vi "RemoveUnexpectedMetrics.vi"(8 "error in (no error)":errorcluster, 9 "Startup Analysis Configuration":T4, 11 "data in":T1) -> (0 "error out":errorcluster)   [LabVIEW 2017, in "McsaStartupAnalysis.lvlib"]
uses:
  <vilib>/addons/InsightCM/Devices/Shared/Mcsa/McsaStartupAnalysis/McsaStartupAnalysis.lvlib
  <vilib>/addons/InsightCM/Devices/Shared/Mcsa/McsaStartupAnalysis/controls/Config.ctl
  <vilib>/addons/InsightCM/Devices/Shared/Mcsa/McsaStartupAnalysis/controls/Group.ctl
  <vilib>/addons/InsightCM/Devices/Shared/Mcsa/McsaStartupAnalysis/controls/ChannelForStartup.ctl
  <vilib>/addons/InsightCM/Devices/Shared/Mcsa/McsaStartupAnalysis/controls/StartupFeature.ctl
  <vilib>/addons/InsightCM/Devices/Shared/Mcsa/McsaStartupAnalysis/controls/MotorInfo.ctl
  <vilib>/addons/InsightCM/Devices/Shared/Common/FileFlow/controls/data_eventRef.ctl
  <vilib>/addons/InsightCM/Devices/Shared/Common/DataEvent/controls/EventReference.ctl
  <vilib>/addons/InsightCM/Devices/Shared/Common/DataEvent/controls/Event.ctl
  <vilib>/addons/InsightCM/MessageBus/Base/controls/DataEvent.ctl
  <vilib>/addons/InsightCM/MessageBus/Base/controls/KeyValuePair.ctl
  <vilib>/addons/InsightCM/Devices/Shared/Common/DataEvent/controls/DataSet.ctl
  <vilib>/addons/InsightCM/MessageBus/Base/controls/DataSetMetadata.ctl
  <vilib>/addons/InsightCM/MessageBus/Base/controls/TrendPoint.ctl
  <vilib>/addons/InsightCM/MessageBus/Base/controls/TrendAlarmUpdate.ctl
  <vilib>/addons/InsightCM/MessageBus/Base/controls/TrendAlarmTransition.ctl
  <vilib>/addons/PointValueMap/controls/PointMap.ctl
  <vilib>/addons/InsightCM/Utilities/PropertyHelpers/PropertyHelpers.lvlib
  <vilib>/addons/InsightCM/Devices/Shared/Common/DataEvent/DataEvent.lvlib
  <vilib>/addons/PointValueMap/PointValueMap.lvlib
  <vilib>/addons/InsightCM/Devices/Shared/Common/FileFlow/FileFlow.lvlib
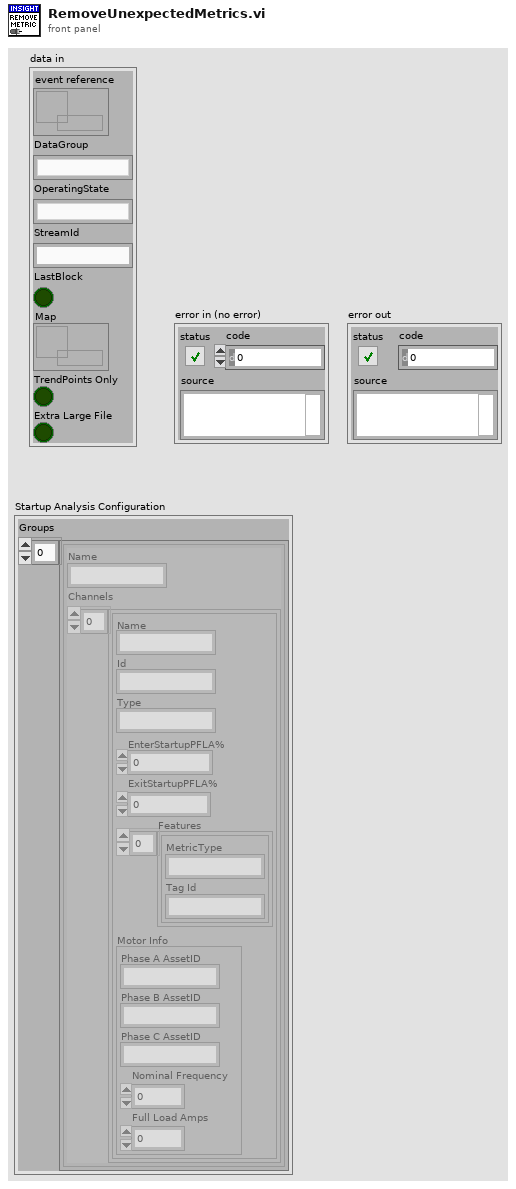
[diagram p1: front panel]
types:
  T1 = typedef "FileFlow.lvlib/data_eventRef.ctl" = cluster{"event reference":T2, "DataGroup":string, "OperatingState":string, "StreamId":string, "LastBlock":bool, "Map":T3, "TrendPoints Only":bool, "Extra Large File":bool}
  T2 = typedef "DataEvent.lvlib/EventReference.ctl" = refnum<data-value>
  T3 = typedef "PointValueMap.lvlib/PointMap.ctl" = refnum<data-value>
  T4 = typedef "McsaStartupAnalysis.lvlib/Config.ctl" = cluster{"Groups":T5[]}
  T5 = typedef "McsaStartupAnalysis.lvlib/Group.ctl" = cluster{"Name":string, "Channels":T6[]}
  T6 = typedef "McsaStartupAnalysis.lvlib/ChannelForStartup.ctl" = cluster{"Name":string, "Id":string, "Type":string, "EnterStartupPFLA%":dbl, "ExitStartupPFLA%":dbl, "Features":T7[], "Motor Info":T8}
  T7 = typedef "McsaStartupAnalysis.lvlib/StartupFeature.ctl" = cluster{"MetricType":string, "Tag Id":string}
  T8 = typedef "McsaStartupAnalysis.lvlib/MotorInfo.ctl" = cluster{"Phase A AssetID":string, "Phase B AssetID":string, "Phase C AssetID":string, "Nominal Frequency":dbl, "Full Load Amps":dbl}
  T9 = typedef "DataEvent.lvlib/Event.ctl" = cluster{"DataEvent":T10, "DataSets":T12[], "TrendPoints":T14[], "Alarms":T15[]}
  T10 = typedef "DataEvent.ctl" = cluster{"Id":string, "AssetNodeId":string, "Timestamp":i64, "Props":T11[]}
  T11 = typedef "KeyValuePair.ctl" = cluster{"Key":string, "Value":string}
  T12 = typedef "DataEvent.lvlib/DataSet.ctl" = cluster{"DataSetMetadata":T13, "Values":sgl[], "Values DVR":refnum<data-value>}
  T13 = typedef "DataSetMetadata.ctl" = cluster{"Id":string, "DataEventId":string, "AssetNodeId":string, "Type":string, "T0":i64, "Props":T11[]}
  T14 = typedef "TrendPoint.ctl" = cluster{"TrendPointId":string, "DataEventId":string, "Timestamp":i64, "Value":dbl, "Props":T11[]}
  T15 = typedef "TrendAlarmUpdate.ctl" = cluster{"RuleId":string, "Transition":T16}
  T16 = typedef "TrendAlarmTransition.ctl" = cluster{"At":i64, "Severity":i32, "Value":dbl}
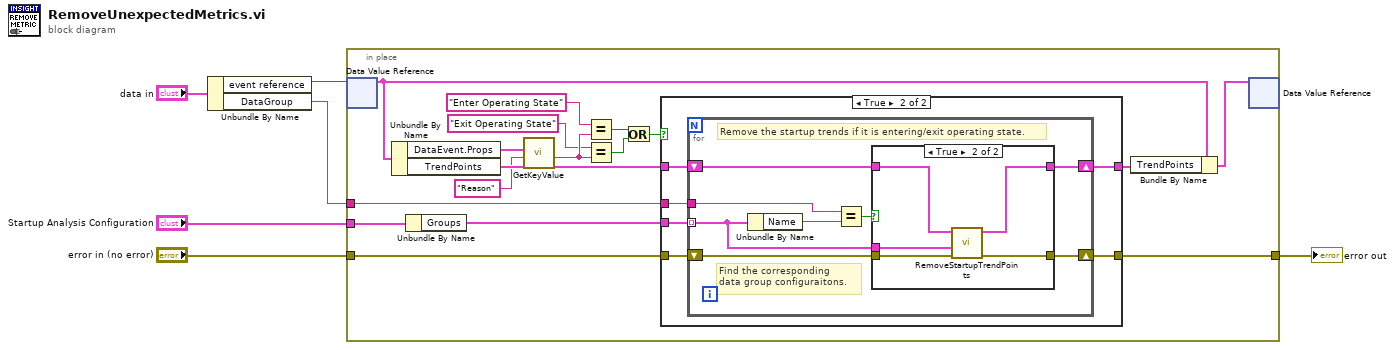
[diagram p0: block diagram]
diagram:
  n1 = Unbundle By Name("data in") -> ("event reference"=w4:T2, "DataGroup"=w3:string)
  n2 = in-place {
    in-place-border: "Startup Analysis Configuration" -> [w22]
    in-place-border: w3 -> [w17]
    in-place-border: "error in (no error)" -> [w16]
    in-place-border: [w15] -> w1
    n3 = in-place-dvr #1(w4) -> (w20:T9)  [unwired: 1 out]
    n4 = Unbundle By Name(w20) -> ("DataEvent.Props"=w14:T11[], "TrendPoints"=w19:T14[])
    n5 = Unbundle By Name(w22) -> ("Groups"=w23:T5[])
    n6 = call <vilib>:"GetKeyValue.vi"("key"="Reason" ("x"), "key value pairs"=w14) -> ("value"=w12:string)  [unwired: 7 in, 2 out]
    n7 = Equal?(x="Enter Operating State", y=w12) -> (x = y?=w9:bool)
    n8 = Equal?(x="Exit Operating State", y=w12) -> (x = y?=w8:bool)
    n9 = Or(x=w9, y=w8) -> (x .or. y?=w7:bool)
    n10 = case shown="True" w7 {
      tunnel: w23 -> [_ w31]
      tunnel: w19 -> [w25 w30]
      tunnel: [w25 w29] -> w18
      tunnel: w17 -> [_ w28]
      tunnel: w16 -> [w24 w27]
      tunnel: [w24 w26] -> w15
      frame False {
        # "Do nothing if it is not entering or exiting the operating state."
      }
      frame True {
        n11 = for {
          tunnel: w31 -> [w37] mode=indexing
          shift-right: [w35] -> w29
          shift-left: w30 -> [w36]
          tunnel: w28 -> [w34]
          shift-right: [w32] -> w26
          shift-left: w27 -> [w33]
          # "Remove the startup trends if it is entering/exit operating state."
          # "Find the corresponding\ndata group configuraitons."
          n12 = Unbundle By Name(w37) -> ("Name"=w39:string)
          n13 = Equal?(x=w34, y=w39) -> (x = y?=w38:bool)
          n14 = case shown="True" w38 {
            tunnel: w37 -> [_ w42]
            tunnel: w36 -> [w41 w46]
            tunnel: [w41 w45] -> w35
            tunnel: w33 -> [w40 w44]
            tunnel: [w40 w43] -> w32
            frame False {
            }
            frame True {
              n15 = call <vilib>:"RemoveStartupTrendPoints.vi"("error in (no error)"=w44, "Group"=w42, "TrendPoints in"=w46) -> ("error out"=w43:errorcluster, "TrendPoints out"=w45:T14[])  [unwired: 7 in]
            }
          }
        }
      }
    }
    n16 = Bundle By Name(cluster=w20, "TrendPoints"=w18) -> (w21:T9)
    n17 = in-place-dvr #1(w21) -> ()  [unwired: 2 out]
  }
  "error out" <- w1
